vi "Agilent 33XXX Series Generate Arbitrary Waveform_AS1.vi"(1 "error in (no error)":errorcluster, 2 "Frequency (1000 Hz)":dbl=1000000.0, 3 "Enum":enum16{"Triangle", "Sine"}(ring)) -> (0 "error out":errorcluster)   [LabVIEW 2016]
doc: "Shows how to configure then create an arbitrary waveform."
uses:
  Instance           2 56Saved   Agilent 33XXX Series Generate Arbitrary Waveform .vi
  Instance           1 56Saved   Agilent 33XXX Series Generate Arbitrary Waveform .vi
  Agilent 33XXX Series.lvlib
panel:
  in  "Serial Configuration":T1={"Baud Rate"=9600, "Parity"=0, "Data Bits"=8, "Flow Control"=4} {"Flow Control" items=["None", "XON/XOFF", "RTS/CTS", "XON/XOFF & RTS/CTS", "DTR/DSR", "XON/XOFF & DTR/DSR"]; "Data Bits" items=["7"=7, "8"=8]; "Parity" items=["None", "Odd", "Even", "Mark", "Space"]; "Baud Rate" items=["300"=300, "600"=600, "1200"=1200, "2400"=2400, "4800"=4800, "9600"=9600, "19200"=19200]}
  in  "VISA resource name":refnum<visa-resource-name>="GPIB0::4::INSTR"
  in  "Gain (1.0)":dbl=2.5
  in  "Offset (0 V)":dbl
  # "(c) 2005 - 2013 National Instruments.  ALL RIGHTS RESERVED."
  # "To edit the Arbitrary Waveform, use the Simulate Arbitrary Signal on the block diagram; or choose from the options below."
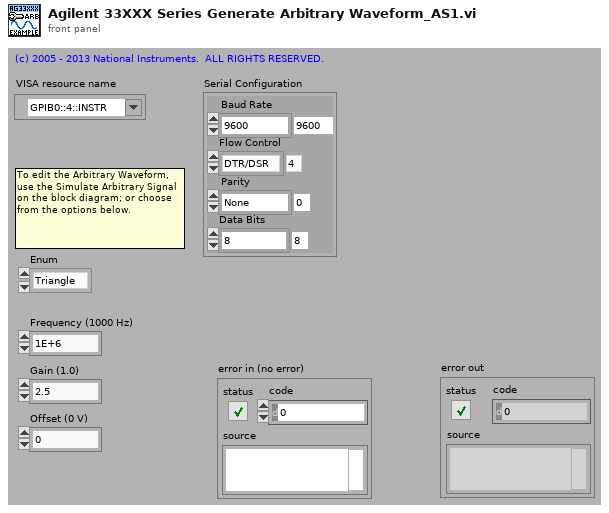
[diagram p1: front panel]
types:
  T1 = cluster{"Baud Rate":u32, "Parity":u16, "Data Bits":u16, "Flow Control":u16}
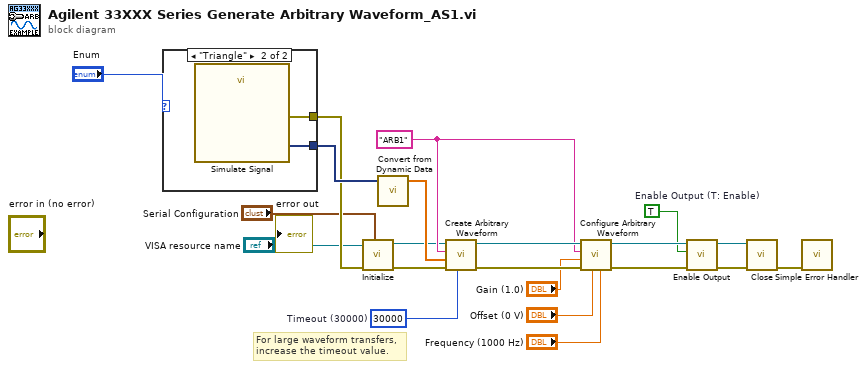
[diagram p0: block diagram]
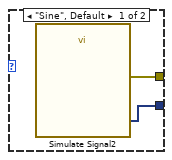
[diagram p2: hidden frame]
diagram:
  w13 = "ARB1" ("Arbitrary Waveform Name")
  w10 = u32 30000  # Timeout (30000)
  w14 = TRUE  # Enable Output (T: Enable)
  # "For large waveform transfers, increase the timeout value."
  n1 = case shown="\"Triangle\"" "Enum" {
    tunnel: [w22 w25] -> w7
    tunnel: [w23 w24] -> w5
    frame "Sine", Default {
      n2 = call "Simulate Signal2"() -> ("Sine"=w22:dynamicdata, "error out"=w23:errorcluster)  [unwired: 14 in]
    }
    frame "Triangle" {
      n3 = call "Simulate Signal"() -> ("Triangle"=w25:dynamicdata, "error out"=w24:errorcluster)  [unwired: 14 in]
    }
  }
  n4 = call "Initialize.vi"("Serial Configuration"="Serial Configuration", "error in (no error)"=w5, "VISA resource name"="VISA resource name") -> ("error out"=w6:errorcluster, "VISA resource name out"=w8:refnum<visa-resource-name>)  [unwired: 7 in]
  n5 = call "Convert from Dynamic Data"("Dynamic Data Type"=w7) -> ("Array"=w9:dbl[])  [unwired: 3 in]
  n6 = call "Create Arbitrary Waveform.vi"("Timeout (10000)"=w10, "error in (no error)"=w6, "Arbitrary Waveform Data"=w9, "Arbitrary Waveform Name (\"ARB1\")"=w13, "VISA resource name"=w8) -> ("error out"=w19:errorcluster, "VISA resource name out"=w20:refnum<visa-resource-name>)  [unwired: 5 in]
  n7 = call "Configure Arbitrary Waveform.vi"("Frequency (1000 Hz)"="Frequency (1000 Hz)", "Offset (0.00 V)"="Offset (0 V)", "error in (no error)"=w19, "Gain (1.0)"="Gain (1.0)", "Arbitrary Waveform Name (\"ARB1\")"=w13, "VISA resource name"=w20) -> ("error out"=w17:errorcluster, "VISA resource name out"=w18:refnum<visa-resource-name>)  [unwired: 4 in]
  n8 = call "Enable Output.vi"("error in (no error)"=w17, "Enable Output  (T: Enable)"=w14, "VISA resource name"=w18) -> ("error out"=w16:errorcluster, "VISA resource name out"=w15:refnum<visa-resource-name>)  [unwired: 7 in]
  n9 = call "Close.vi"("error in (no error)"=w16, "VISA resource name"=w15) -> ("error out"=w21:errorcluster)  [unwired: 9 in]
  n10 = call <vilib>:"Simple Error Handler.vi"("error in (no error)"=w21) -> ()  [unwired: 4 in, 5 out]
